vi "index helper.vi"(9 "last index":i32=-1, 10 "this index":i32=-1) -> (1 "next index":i32)   [LabVIEW 2015, in "Index JSON Array.xnode"]
uses:
  Index JSON Array.xnode
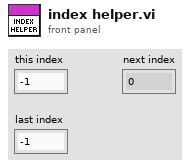
[diagram p1: front panel]
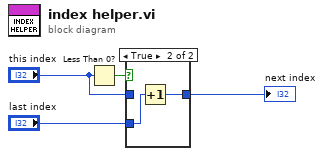
[diagram p0: block diagram]
diagram:
  n1 = Less Than 0?(x="this index") -> (x < 0?=w4:bool)
  n2 = case shown="True" w4 {
    tunnel: [w5 w6] -> w1
    tunnel: "this index" -> [w5 _]
    tunnel: "last index" -> [_ w7]
    frame False {
    }
    frame True {
      n3 = Increment(x=w7) -> (x+1=w6:i32)
    }
  }
  "next index" <- w1
